vi "Untitled 1.vi"() -> ()   [LabVIEW 2025]
uses:
  <vilib>/DAQmx/read.llb/DAQmx Read (Counter U32 1Chan 1Samp).vi
  <vilib>/DAQmx/read.llb/DAQmx Read (Analog Wfm 1Chan NSamp).vi
  <vilib>/DAQmx/create/channels.llb/DAQmx Create Channel (AI-Voltage-Basic).vi
  <vilib>/DAQmx/configure/timing.llb/DAQmx Timing (Sample Clock).vi
  <vilib>/DAQmx/create/channels.llb/DAQmx Create Channel (CI-Count Edges).vi
  <vilib>/DAQmx/miscellaneous.llb/DAQmx Fill In Error Info.vi
  <vilib>/DAQmx/create/channels.llb/DAQmx Create Channel (CO-Pulse Generation-Frequency).vi
  <vilib>/DAQmx/configure/timing.llb/DAQmx Timing (Implicit).vi
  <vilib>/Waveform/WDTFileIO.llb/Export Waveform To Spreadsheet File.vi
  <resource>/objmgr/daqmx.rc
panel:
  in  "append to file? (new file:F)":bool=TRUE
  in  "Path":path
  in  "stop":bool
  in  "Pulso":tag
  in  "stop 2":bool
  out "Numeric":i32
  out "Waveform Graph":waveform(dbl)(graph)
  out "data":u32
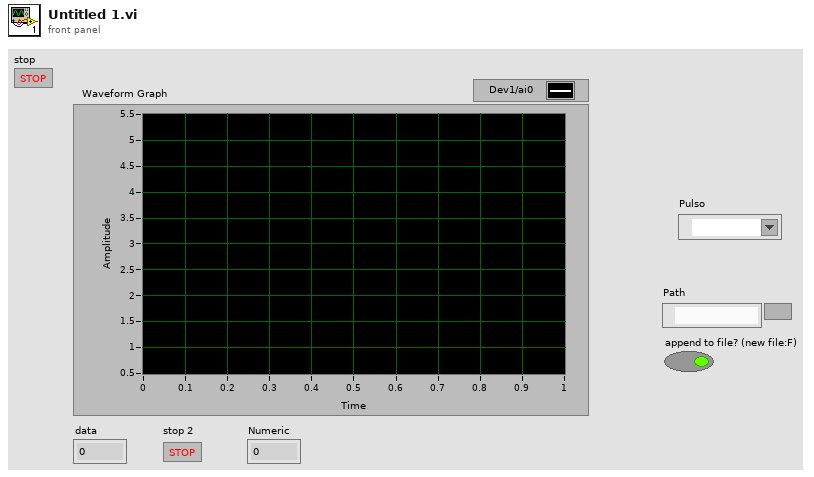
[diagram p1: front panel]
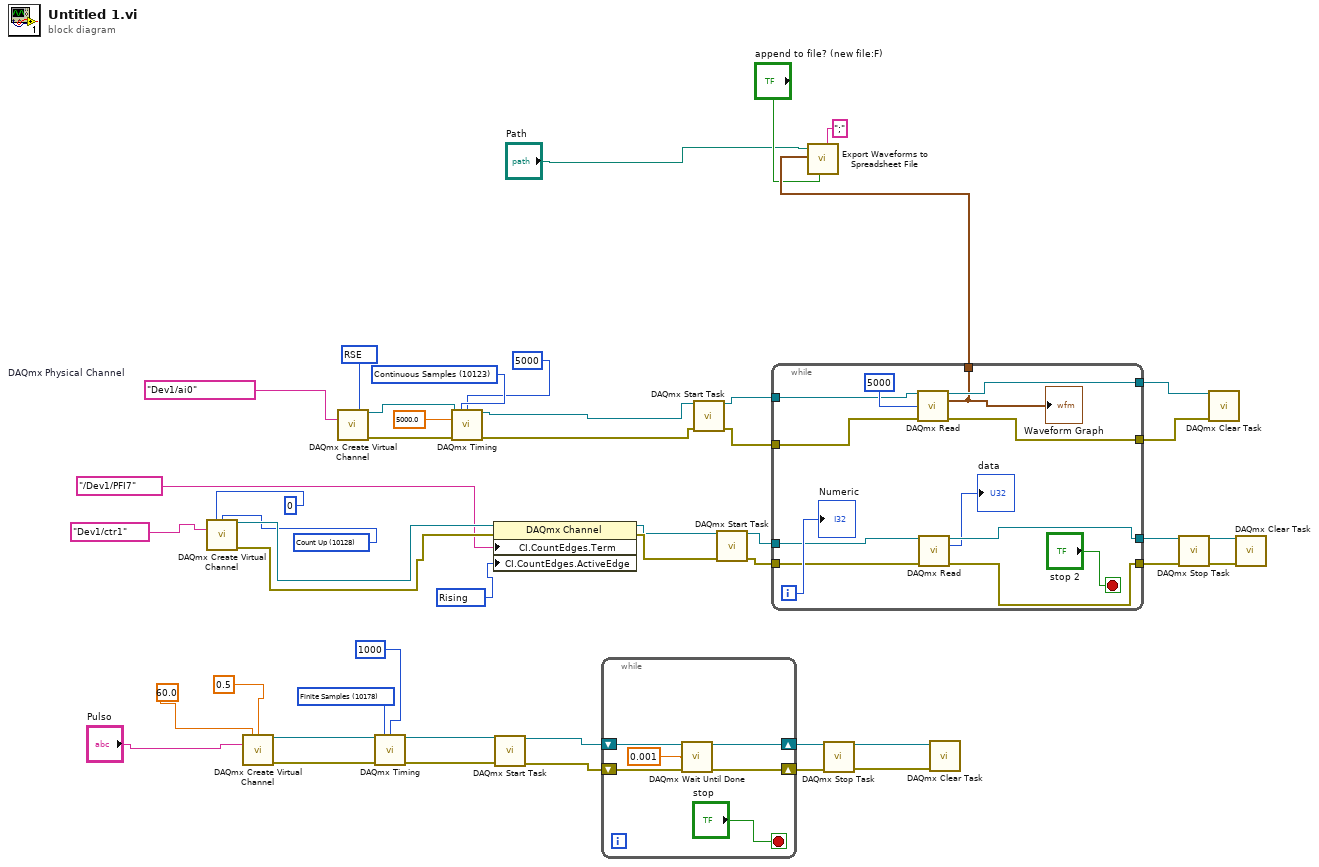
[diagram p0: block diagram]
diagram:
  w19 = 10178 items=["Finite Samples"=10178, "Continuous Samples"=10123, "Hardware Timed Single Point"=12522] ("sample mode")
  w29 = 10280 items=["Rising"=10280, "Falling"=10171] ("CI.CountEdges.ActiveEdge")
  w27 = 10128 items=["Count Up"=10128, "Count Down"=10124, "Externally Controlled"=10326] ("count direction")
  w23 = 10083 items=["Default"=-1, "RSE"=10083, "NRSE"=10078, "Differential"=10106, "Pseudodifferential"=12529] ("input terminal configuration")
  w26 = 10123 items=["Finite Samples"=10178, "Continuous Samples"=10123, "Hardware Timed Single Point"=12522] ("sample mode")
  w22 = tag "Dev1/ai0"  # DAQmx Physical Channel
  n1 = call-poly <vilib>:"DAQmx Create Virtual Channel.vi"("initial count"=u32 0, "count direction"=w27, "counter"=tag "Dev1/ctr1") -> ("task out"=w38:refnum<k21>, "error out"=w39:errorcluster)  [unwired: 11 in]
  n2 = call-poly <vilib>:"DAQmx Create Virtual Channel.vi"("frequency"=60.0 ("Frequência"), "duty cycle"=0.5, "counter"="Pulso") -> ("task out"=w21:refnum<k21>, "error out"=w20:errorcluster)  [unwired: 11 in]
  n3 = call-poly <vilib>:"DAQmx Create Virtual Channel.vi"("input terminal configuration"=w23, "physical channels"=w22) -> ("task out"=w31:refnum<k21>, "error out"=w32:errorcluster)  [unwired: 12 in]
  n4 = call-poly <vilib>:"DAQmx Timing.vi"("task/channels in"=w21, "sample mode"=w19, "samples per channel"=1000, "error in"=w20) -> ("task out"=w15:refnum<k21>, "error out"=w14:errorcluster)  [unwired: 10 in]
  n5 = call-poly <vilib>:"DAQmx Timing.vi"("task/channels in"=w31, "sample mode"=w26, "samples per channel"=5000, "rate"=5000.0, "error in"=w32) -> ("task out"=w36:refnum<k21>, "error out"=w37:errorcluster)  [unwired: 9 in]
  n6 = property class="DAQmx Channel"(reference=w38, error in=w39, "CI.CountEdges.Term"=tag "/Dev1/PFI7", "CI.CountEdges.ActiveEdge"=w29) -> (reference out=w40:refnum<k21>, error out=w41:errorcluster)
  n7 = call <vilib>:"DAQmx Start Task.vi"("task/channels in"=w15, "error in"=w14) -> ("task out"=w13:refnum<k21>, "error out"=w12:errorcluster)  [unwired: 12 in]
  n8 = while {
    shift-right: [w51] -> w11
    shift-left: w13 -> [w53]
    shift-right: [w50] -> w10
    shift-left: w12 -> [w52]
    stop <- "stop" stop-if-true
    n9 = call <vilib>:"DAQmx Wait Until Done.vi"("task/channels in"=w53, "timeout (sec)"=0.001, "error in"=w52) -> ("task out"=w51:refnum<k21>, "error out"=w50:errorcluster)  [unwired: 11 in]
  }
  n10 = call <vilib>:"DAQmx Start Task.vi"("task/channels in"=w36, "error in"=w37) -> ("task out"=w34:refnum<k21>, "error out"=w35:errorcluster)  [unwired: 12 in]
  n11 = call <vilib>:"DAQmx Start Task.vi"("task/channels in"=w40, "error in"=w41) -> ("task out"=w42:refnum<k21>, "error out"=w43:errorcluster)  [unwired: 12 in]
  n12 = while {
    tunnel: [w65] -> w33
    tunnel: [w66] -> w30
    tunnel: w34 -> [w61]
    tunnel: w35 -> [w60]
    tunnel: w42 -> [w59]
    tunnel: w43 -> [w58]
    tunnel: [w57] -> w46
    tunnel: [w56] -> w47
    tunnel: [w54] -> w5
    i -> [w62]
    stop <- "stop 2" stop-if-true
    n13 = call-poly <vilib>:"DAQmx Read.vi"("task/channels in"=w61, "number of samples per channel"=5000, "error in"=w60) -> ("task out"=w66:refnum<k21>, "data"=w54:waveform(dbl), "error out"=w65:errorcluster)  [unwired: 10 in]
    "Waveform Graph" <- w54
    n14 = call-poly <vilib>:"DAQmx Read.vi"("task/channels in"=w59, "error in"=w58) -> ("task out"=w57:refnum<k21>, "data"=→"data":u32, "error out"=w56:errorcluster)  [unwired: 11 in]
    "Numeric" <- w62
  }
  n15 = call-poly <vilib>:"Export Waveforms to Spreadsheet File.vi"("delimiter (Tab)"=";", "append to file? (new file:F)"="append to file? (new file:F)", "waveform"=w5, "file path (dialog if empty)"="Path") -> ()  [unwired: 6 in, 2 out]
  n16 = call <vilib>:"DAQmx Stop Task.vi"("task/channels in"=w11, "error in"=w10) -> ("task out"=w9:refnum<k21>, "error out"=w8:errorcluster)  [unwired: 12 in]
  n17 = call <vilib>:"DAQmx Clear Task.vi"("task in"=w9, "error in"=w8) -> ()  [unwired: 13 in, 1 out]
  n18 = call <vilib>:"DAQmx Stop Task.vi"("task/channels in"=w46, "error in"=w47) -> ("task out"=w44:refnum<k21>, "error out"=w45:errorcluster)  [unwired: 12 in]
  n19 = call <vilib>:"DAQmx Clear Task.vi"("task in"=w30, "error in"=w33) -> ()  [unwired: 13 in, 1 out]
  n20 = call <vilib>:"DAQmx Clear Task.vi"("task in"=w44, "error in"=w45) -> ()  [unwired: 13 in, 1 out]
